vi "Postset Then.vi"(8 "error in (no error)":errorcluster) -> (0 "error out":errorcluster)   [LabVIEW 2017, in "Unit Tests.lvlib"]
uses:
  Unit Tests.lvlib
  Promise Future/Future/Future.lvclass/Future.ctl
  3ca253fc-3f3c-47f3-9a24-db5028bdb027.vi
  8ac51386-f088-464e-addd-59ca3964afbe.vi
  95dc31ad-9ffa-4fc7-be26-3e0641f1d074.vi
  b2e5f197-10a3-4ad7-b26c-b44c03cc53a7.vi
  Promise Future/Future/Then.vi
  Promise Future/Promise/Promise.lvclass
  E:/Promise/Promise Future/Future/Future.lvclass
  Promise Future/Promise/Read Future.vi
  Basic Then Callback.vi
  Promise Future/Future/VI Name Wrapper.vi
  Promise Future/State/Then.vi
  Promise Future/Future/Fulfull (Value).vi
  Promise Future/Future/Read Value (private).vi
  Promise Future/Future/Future.lvclass
  <vilib>/addons/_JKI Toolkits/Caraya/classes/Test/Test.lvclass
  <vilib>/addons/_JKI Toolkits/Caraya/classes/Assert/Assert.lvclass
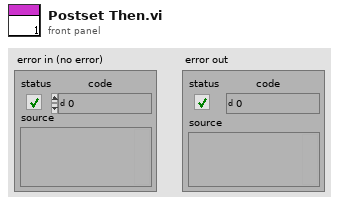
[diagram p1: front panel]
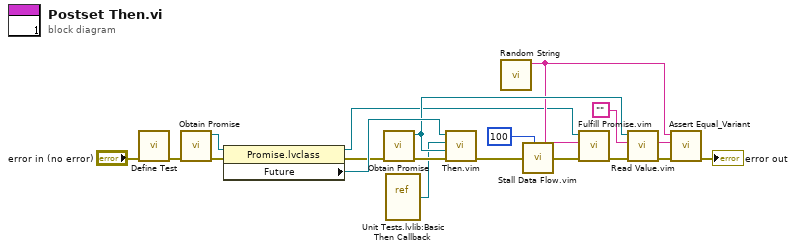
[diagram p0: block diagram]
diagram:
  n1 = call <vilib>:"Define Test.vi"("error in (no error)"="error in (no error)") -> ("error out"=w13:errorcluster)  [unwired: 10 in]
  n2 = call "Obtain Promise.vi"("error in (no error)"=w13) -> ("error out"=w6:errorcluster, "Promise out"=w7:refnum<class "Promise.lvclass">)  [unwired: 8 in, 1 out]
  n3 = property class="Promise.lvclass"(reference=w7, error in=w6) -> (reference out=w3:refnum<class "Promise.lvclass">, error out=w14:errorcluster, "Future"=w19:refnum<class "Future.lvclass">)
  n4 = call "Obtain Promise.vi"("error in (no error)"=w14) -> ("error out"=w15:errorcluster, "Promise out"=w11:refnum<class "Promise.lvclass">)  [unwired: 8 in, 1 out]
  n5 = vi-ref "Unit Tests.lvlib:Basic Then Callback.vi"() -> (w8:refnum<vi>)
  n6 = call "Then.vim"("error in (no error)"=w15, "Scope"=w11, "Callback"=w8, "Future in"=w19) -> ("error out"=w5:errorcluster)  [unwired: 6 in, 1 out]
  n7 = call "Random String.vi"() -> ("string"=w9:string)  [unwired: 11 in]
  n8 = call "Stall Data Flow.vim"("value in"=w5, "milliseconds to wait"=u32 100) -> ("value out"=w2:errorcluster)  [unwired: 1 out]
  n9 = call "Fulfill Promise.vim"("error in (no error)"=w2, "Value"=w9, "Promise in"=w3) -> ("error out"=w4:errorcluster)  [unwired: 7 in, 1 out]
  n10 = call "Read Value.vim"("error in (no error)"=w4, "Default Value"="", "Future in"=w11) -> ("error out"=w17:errorcluster, "Value"=w10:string)  [unwired: 5 in, 2 out]
  n11 = call <vilib>:"Assert Equal_Variant.vi"("error in (no error)"=w17, "Y"=w10, "X"=w9) -> ("error out"=→"error out":errorcluster)  [unwired: 8 in]
